vi "Set Operator.vi"(11 "Config Cluster Version":string) -> ()   [LabVIEW 2015, in "Tool Cfg.lvlib"]
uses:
  Tool Cfg.lvlib
  ConfigGLOB.vi
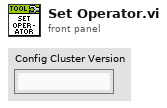
[diagram p1: front panel]
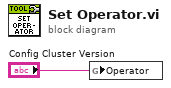
[diagram p0: block diagram]
diagram:
  n1 = global write "ConfigGLOB.vi" "Operator"("Config Cluster Version") -> ()
